vi "Connect.vi"(8 "error in":errorcluster, 11 "PIOD in":refnum<class "PIOD.lvclass">) -> (0 "error out":errorcluster, 3 "PIOD out":refnum<class "PIOD.lvclass">)   [LabVIEW 2018, in "PIOD.lvlib" / "PIOD.lvclass"]
uses:
  PIOD.lvclass
  PIOD.lvclass/PIOD.ctl
  PPLs/Configuration/Configuration.lvlibp/Configuration.lvclass
  PPLs/PLC/Parent/PLC.lvlibp/PLC.lvclass
  C:/AME Test Engineering/LabVIEW/PPLs/PLC/Parent/PLC.lvlibp/PLC.lvclass
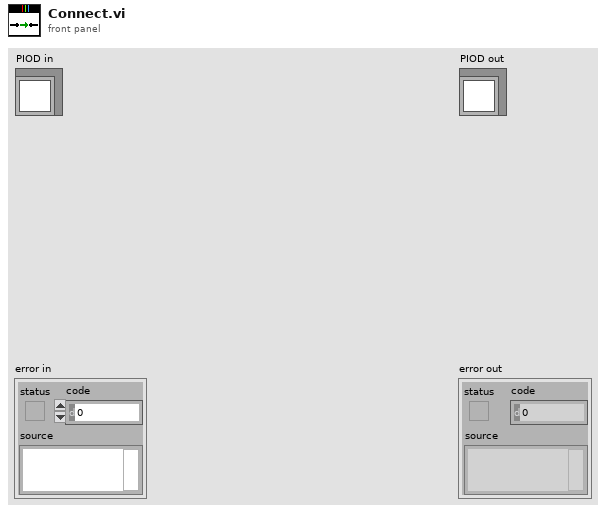
[diagram p1: front panel]
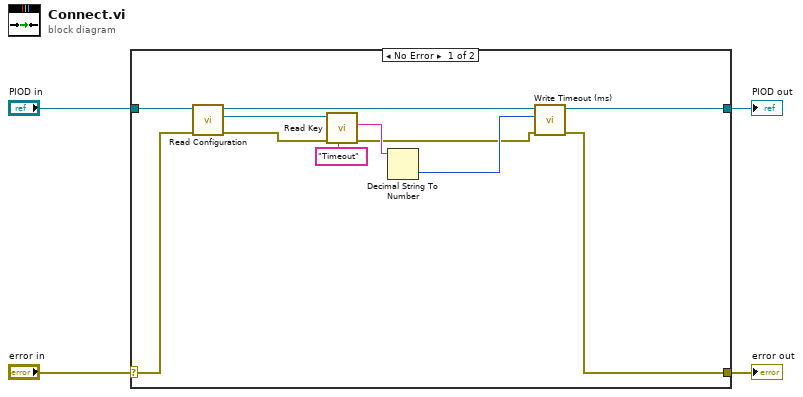
[diagram p0: block diagram]
diagram:
  n1 = case shown="No Error" "error in" {
    selector: "error in" -> [w12 w17]
    tunnel: [w5 w17] -> w3
    tunnel: [w8 w16] -> w1
    tunnel: "PIOD in" -> [w13 w16]
    frame No Error {
      n2 = call "Read Configuration.vi"("error in (no error)"=w12, "PLC in"=w13) -> ("error out"=w11:errorcluster, "Configuration"=w10:refnum<class "Configuration.lvclass">, "PLC out"=w9:refnum<class "PIOD.lvclass">)  [unwired: 7 in]
      n3 = call "Read Key.vi"("Key:"="Timeout", "error in"=w11, "Configuration in"=w10) -> ("error out"=w6:errorcluster, "Value"=w14:string)  [unwired: 6 in, 1 out]
      n4 = Decimal String To Number(string=w14) -> (number=w7:i32)  [unwired: 2 in, 1 out]
      n5 = call "Write Timeout (ms).vi"("error in (no error)"=w6, "Timeout (ms)"=w7, "PIOD in"=w9) -> ("error out"=w5:errorcluster, "PIOD out"=w8:refnum<class "PIOD.lvclass">)  [unwired: 7 in]
    }
    frame Error {
    }
  }
  "error out" <- w3
  "PIOD out" <- w1
